vi "SR_M_Resize_Image.vi"(9 "New Width (pixels)":i32=1020, 10 "New Height (pixels)":i32=1020, 11 "image data in":T1) -> (3 "image data out":T1)   [LabVIEW 2015, in "Shore Library.lvlib"]
uses:
  Shore Library.lvlib
  <vilib>/picture/picture.llb/imagedata.ctl
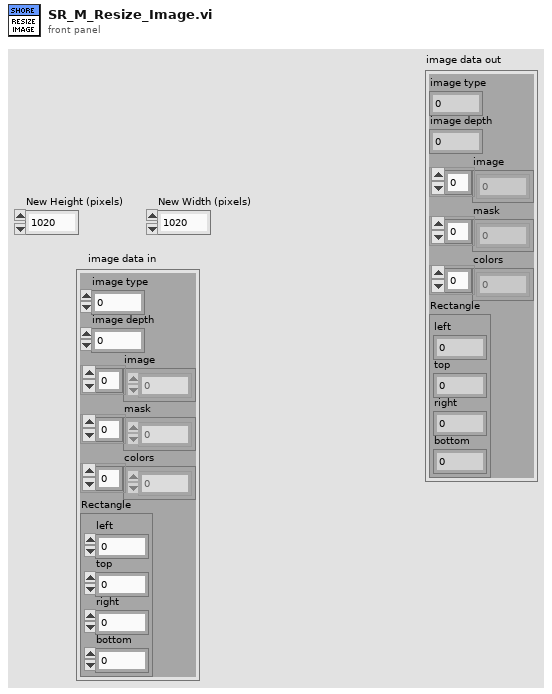
[diagram p1: front panel]
types:
  T1 = typedef "imagedata.ctl" = cluster{"image type":i32, "image depth":i32, "image":u8[], "mask":u8[], "colors":u32[], "Rectangle":cluster{"left":i16, "top":i16, "right":i16, "bottom":i16}}
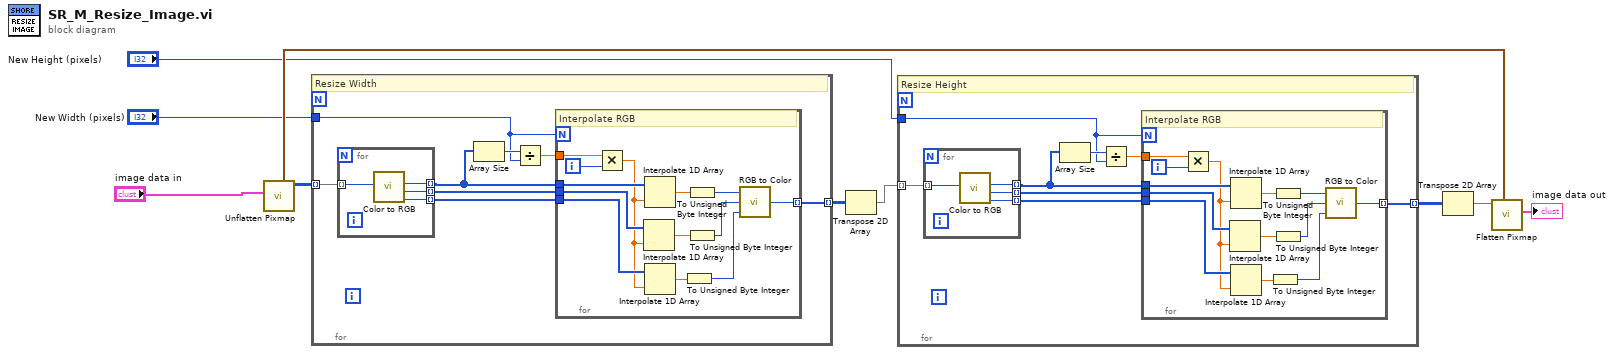
[diagram p0: block diagram]
diagram:
  n1 = call <vilib>:"Unflatten Pixmap.vi"("image data"="image data in") -> ("24-bit pixmap"=w10:u32[][], "top left"=w9:cluster{"x":i16, "y":i16})  [unwired: 4 in, 5 out]
  n2 = for {
    tunnel: w10 -> [w17] mode=indexing
    tunnel: [w12] -> w7 mode=indexing
    tunnel: "New Width (pixels)" -> [w11]
    # "Resize Width"
    n3 = for {
      tunnel: w17 -> [w22] mode=indexing
      tunnel: [w21] -> w16 mode=indexing
      tunnel: [w20] -> w14 mode=indexing
      tunnel: [w19] -> w13 mode=indexing
      n4 = call <vilib>:"Color to RGB.vi"("Color"=w22) -> ("R"=w21:u8, "G"=w20:u8, "B"=w19:u8)  [unwired: 1 out]
    }
    n5 = Array Size(array=w16) -> (size(s)=w18:i32)
    n6 = Divide(x=w18, y=w11) -> (x/y=w15:dbl)
    n7 = for {
      N: w11 -> [_]
      tunnel: w16 -> [w35]
      tunnel: w15 -> [w33]
      tunnel: w14 -> [w30]
      tunnel: w13 -> [w29]
      tunnel: [w23] -> w12 mode=indexing
      i -> [w34]
      # "Interpolate RGB"
      n8 = Multiply(x=w33, y=w34) -> (x*y=w28:dbl)
      n9 = Interpolate 1D Array(1:w28, 2:w30) -> (0:w32:dbl)
      n10 = Interpolate 1D Array(1:w28, 2:w35) -> (0:w27:dbl)
      n11 = Interpolate 1D Array(1:w28, 2:w29) -> (0:w31:dbl)
      n12 = To Unsigned Byte Integer(number=w31) -> (unsigned 8bit integer=w24:u8)
      n13 = To Unsigned Byte Integer(number=w27) -> (unsigned 8bit integer=w26:u8)
      n14 = To Unsigned Byte Integer(number=w32) -> (unsigned 8bit integer=w25:u8)
      n15 = call <vilib>:"RGB to Color.vi"("B"=w24, "G"=w25, "R"=w26) -> ("Color"=w23:u32)
    }
  }
  n16 = Transpose 2D Array(2D array=w7) -> (transposed array=w6:u32[][])
  n17 = for {
    tunnel: w6 -> [w42] mode=indexing
    tunnel: [w37] -> w4 mode=indexing
    tunnel: "New Height (pixels)" -> [w36]
    # "Resize Height"
    n18 = for {
      tunnel: w42 -> [w47] mode=indexing
      tunnel: [w46] -> w41 mode=indexing
      tunnel: [w45] -> w39 mode=indexing
      tunnel: [w44] -> w38 mode=indexing
      n19 = call <vilib>:"Color to RGB.vi"("Color"=w47) -> ("R"=w46:u8, "G"=w45:u8, "B"=w44:u8)  [unwired: 1 out]
    }
    n20 = Array Size(array=w41) -> (size(s)=w43:i32)
    n21 = Divide(x=w43, y=w36) -> (x/y=w40:dbl)
    n22 = for {
      N: w36 -> [_]
      tunnel: w41 -> [w60]
      tunnel: w40 -> [w58]
      tunnel: w39 -> [w55]
      tunnel: w38 -> [w54]
      tunnel: [w48] -> w37 mode=indexing
      i -> [w59]
      # "Interpolate RGB"
      n23 = Multiply(x=w58, y=w59) -> (x*y=w53:dbl)
      n24 = Interpolate 1D Array(1:w53, 2:w55) -> (0:w57:dbl)
      n25 = Interpolate 1D Array(1:w53, 2:w60) -> (0:w52:dbl)
      n26 = Interpolate 1D Array(1:w53, 2:w54) -> (0:w56:dbl)
      n27 = To Unsigned Byte Integer(number=w56) -> (unsigned 8bit integer=w49:u8)
      n28 = To Unsigned Byte Integer(number=w52) -> (unsigned 8bit integer=w51:u8)
      n29 = To Unsigned Byte Integer(number=w57) -> (unsigned 8bit integer=w50:u8)
      n30 = call <vilib>:"RGB to Color.vi"("B"=w49, "G"=w50, "R"=w51) -> ("Color"=w48:u32)
    }
  }
  n31 = Transpose 2D Array(2D array=w4) -> (transposed array=w3:u32[][])
  n32 = call <vilib>:"Flatten Pixmap.vi"("top left"=w9, "24-bit pixmap"=w3) -> ("image data"=→"image data out":T1)  [unwired: 9 in]
